vi "S4GUI.vi"(7 "Tab ObsEng":enum32{"Obs", "CCD modes", "Guider", "Eng"}(tab)) -> ()   [LabVIEW 2018] (continued)
            n3354 = call "Write AcquisitionB.vi"("error in (no error)"=w7300, "Acquisition.lvclass"=w7299, "S4ACS_GUI in"=w7297) -> ("error out"=w7303:errorcluster, "S4ACS_GUI out"=w7304:refnum<class "S4GUI.lvclass">)  [unwired: 7 in]
          }
          frame #2 {
            # "object"
            # "suffix"
            # "obsType"
            n3355 = call-dynamic "Read AcquisitionC.vi"("error in (no error)"=w7354, "S4ACS_GUI in"=w7355) -> ("error out"=w7347:errorcluster, "Acquisition.lvclass"=w7346:refnum<class "Acquisition.lvclass">, "S4ACS_GUI out"=w7341:refnum<class "S4GUI.lvclass">)  [unwired: 7 in]
            n3356 = call-dynamic "Read Channel.vi"("error in (no error)"=w7347, "Acquisition in"=w7346) -> ("error out"=w7320:errorcluster, "Channel.lvclass"=w7322:refnum<class "Channel.lvclass">, "Acquisition out"=w7340:refnum<class "Acquisition.lvclass">)  [unwired: 7 in]
            n3357 = local read "Filter3"() -> (w7323:u8)
            n3358 = call-dynamic "Write Filter.vi"("error in (no error)"=w7320, "Filter"=w7323, "Channel in"=w7322) -> ("error out"=w7319:errorcluster, "Channel out"=w7321:refnum<class "Channel.lvclass">)  [unwired: 7 in]
            n3359 = call-dynamic "Read Interface.vi"("error in (no error)"=w7319, "Channel in"=w7321) -> ("error out"=w7332:errorcluster, "Interface.lvclass"=w7333:refnum<class "Interface.lvclass">, "Channel out"=w7345:refnum<class "Channel.lvclass">)  [unwired: 7 in]
            n3360 = call-dynamic "Write Suffix.vi"("error in (no error)"=w7332, "Suffix"=w7351, "Interface in"=w7333) -> ("error out"=w7350:errorcluster, "Interface out"=w7344:refnum<class "Interface.lvclass">)  [unwired: 7 in]
            n3361 = call-dynamic "Write ObsType.vi"("error in (no error)"=w7350, "ObsType"=w7336, "Interface in"=w7344) -> ("error out"=w7349:errorcluster, "Interface out"=w7343:refnum<class "Interface.lvclass">)  [unwired: 7 in]
            n3362 = call-dynamic "Write Object.vi"("error in (no error)"=w7349, "Object"=w7335, "Interface in"=w7343) -> ("error out"=w7348:errorcluster, "Interface out"=w7342:refnum<class "Interface.lvclass">)  [unwired: 7 in]
            n3363 = call-dynamic "Write Comments.vi"("error in (no error)"=w7348, "Comments"=w7337, "Interface in"=w7342) -> ("error out"=w7329:errorcluster, "Interface out"=w7328:refnum<class "Interface.lvclass">)  [unwired: 7 in]
            n3364 = call-dynamic "Write Observer.vi"("error in (no error)"=w7329, "Observer"=w7334, "Interface in"=w7328) -> ("error out"=w7330:errorcluster, "Interface out"=w7331:refnum<class "Interface.lvclass">)  [unwired: 7 in]
            n3365 = call-dynamic "Write Interface.vi"("error in (no error)"=w7330, "Interface.lvclass"=w7331, "Channel in"=w7345) -> ("error out"=w7326:errorcluster, "Channel out"=w7327:refnum<class "Channel.lvclass">)  [unwired: 7 in]
            n3366 = disable-structure shown="Enabled" {
              disable-tunnel: w7327 -> [w7362 w7367]
              disable-tunnel: w7326 -> [w7361 w7366]
              disable-tunnel: [w7359 w7367] -> w7325
              disable-tunnel: [w7356 w7366] -> w7324
              frame Disabled {
                n3367 = call-dynamic "Read State Machine.vi"("error in (no error)"=w7361, "Device in"=w7362) -> ("error out"=w7365:errorcluster, "State Machine.lvclass"=w7358:refnum<class "State Machine.lvclass">, "Device out"=w7360:refnum<class "Channel.lvclass">)  [unwired: 7 in]
                n3368 = call "Next State.vi"("error in (no error)"=w7365, "New_State"=12, "State Machine in"=w7358) -> ("error out"=w7364:errorcluster, "State Machine out"=w7357:refnum<class "State Machine.lvclass">)  [unwired: 7 in]
                n3369 = call-dynamic "Write State Machine.vi"("error in (no error)"=w7364, "State Machine.lvclass"=w7357, "Device in"=w7360) -> ("error out"=w7356:errorcluster, "Device out"=w7359:refnum<class "Channel.lvclass">)  [unwired: 7 in]
              }
              frame Enabled {
              }
            }
            n3370 = call-dynamic "Write Channel.vi"("error in (no error)"=w7324, "Channel.lvclass"=w7325, "Acquisition in"=w7340) -> ("error out"=w7338:errorcluster, "Acquisition out"=w7339:refnum<class "Acquisition.lvclass">)  [unwired: 7 in]
            n3371 = call-dynamic "Write AcquisitionC.vi"("error in (no error)"=w7338, "Acquisition.lvclass"=w7339, "S4ACS_GUI in"=w7341) -> ("error out"=w7352:errorcluster, "S4ACS_GUI out"=w7353:refnum<class "S4GUI.lvclass">)  [unwired: 7 in]
          }
          frame #3 {
            # "object"
            # "suffix"
            # "obsType"
            n3372 = call-dynamic "Read AcquisitionD.vi"("error in (no error)"=w7403, "S4ACS_GUI in"=w7404) -> ("error out"=w7396:errorcluster, "Acquisition.lvclass"=w7395:refnum<class "Acquisition.lvclass">, "S4ACS_GUI out"=w7390:refnum<class "S4GUI.lvclass">)  [unwired: 7 in]
            n3373 = call-dynamic "Read Channel.vi"("error in (no error)"=w7396, "Acquisition in"=w7395) -> ("error out"=w7369:errorcluster, "Channel.lvclass"=w7371:refnum<class "Channel.lvclass">, "Acquisition out"=w7389:refnum<class "Acquisition.lvclass">)  [unwired: 7 in]
            n3374 = local read "Filter4"() -> (w7372:u8)
            n3375 = call-dynamic "Write Filter.vi"("error in (no error)"=w7369, "Filter"=w7372, "Channel in"=w7371) -> ("error out"=w7368:errorcluster, "Channel out"=w7370:refnum<class "Channel.lvclass">)  [unwired: 7 in]
            n3376 = call-dynamic "Read Interface.vi"("error in (no error)"=w7368, "Channel in"=w7370) -> ("error out"=w7381:errorcluster, "Interface.lvclass"=w7382:refnum<class "Interface.lvclass">, "Channel out"=w7394:refnum<class "Channel.lvclass">)  [unwired: 7 in]
            n3377 = call-dynamic "Write Suffix.vi"("error in (no error)"=w7381, "Suffix"=w7400, "Interface in"=w7382) -> ("error out"=w7399:errorcluster, "Interface out"=w7393:refnum<class "Interface.lvclass">)  [unwired: 7 in]
            n3378 = call-dynamic "Write ObsType.vi"("error in (no error)"=w7399, "ObsType"=w7385, "Interface in"=w7393) -> ("error out"=w7398:errorcluster, "Interface out"=w7392:refnum<class "Interface.lvclass">)  [unwired: 7 in]
            n3379 = call-dynamic "Write Object.vi"("error in (no error)"=w7398, "Object"=w7384, "Interface in"=w7392) -> ("error out"=w7397:errorcluster, "Interface out"=w7391:refnum<class "Interface.lvclass">)  [unwired: 7 in]
            n3380 = call-dynamic "Write Comments.vi"("error in (no error)"=w7397, "Comments"=w7386, "Interface in"=w7391) -> ("error out"=w7380:errorcluster, "Interface out"=w7379:refnum<class "Interface.lvclass">)  [unwired: 7 in]
            n3381 = call-dynamic "Write Observer.vi"("error in (no error)"=w7380, "Observer"=w7383, "Interface in"=w7379) -> ("error out"=w7378:errorcluster, "Interface out"=w7377:refnum<class "Interface.lvclass">)  [unwired: 7 in]
            n3382 = call-dynamic "Write Interface.vi"("error in (no error)"=w7378, "Interface.lvclass"=w7377, "Channel in"=w7394) -> ("error out"=w7374:errorcluster, "Channel out"=w7376:refnum<class "Channel.lvclass">)  [unwired: 7 in]
            n3383 = disable-structure shown="Enabled" {
              disable-tunnel: w7376 -> [w7411 w7416]
              disable-tunnel: [w7409 w7416] -> w7375
              disable-tunnel: w7374 -> [w7408 w7415]
              disable-tunnel: [w7407 w7415] -> w7373
              frame Disabled {
                n3384 = call-dynamic "Read State Machine.vi"("error in (no error)"=w7408, "Device in"=w7411) -> ("error out"=w7414:errorcluster, "State Machine.lvclass"=w7406:refnum<class "State Machine.lvclass">, "Device out"=w7410:refnum<class "Channel.lvclass">)  [unwired: 7 in]
                n3385 = call "Next State.vi"("error in (no error)"=w7414, "New_State"=12, "State Machine in"=w7406) -> ("error out"=w7413:errorcluster, "State Machine out"=w7405:refnum<class "State Machine.lvclass">)  [unwired: 7 in]
                n3386 = call-dynamic "Write State Machine.vi"("error in (no error)"=w7413, "State Machine.lvclass"=w7405, "Device in"=w7410) -> ("error out"=w7407:errorcluster, "Device out"=w7409:refnum<class "Channel.lvclass">)  [unwired: 7 in]
              }
              frame Enabled {
              }
            }
            n3387 = call-dynamic "Write Channel.vi"("error in (no error)"=w7373, "Channel.lvclass"=w7375, "Acquisition in"=w7389) -> ("error out"=w7387:errorcluster, "Acquisition out"=w7388:refnum<class "Acquisition.lvclass">)  [unwired: 7 in]
            n3388 = call-dynamic "Write AcquisitionD.vi"("error in (no error)"=w7387, "Acquisition.lvclass"=w7388, "S4ACS_GUI in"=w7390) -> ("error out"=w7401:errorcluster, "S4ACS_GUI out"=w7402:refnum<class "S4GUI.lvclass">)  [unwired: 7 in]
          }
        }
      }
      event "DFLAT Comments", "SFLAT Comments", "DARK Comments", "ZERO Comments", "FOCUS Comments", "OBJECT Comments": Value Change {
        n3389 = event-data() -> ("NewVal"=w7417:string)  [unwired: 1 in, 5 out]
        n3390 = disable-structure shown="Enabled" {
          disable-tunnel: w7425 -> [w7434 w7608]
          disable-tunnel: w7424 -> [w7433 w7607]
          disable-tunnel: w7423 -> [w7432 _]
          disable-tunnel: w7422 -> [w7431 _]
          disable-tunnel: w7421 -> [w7430 _]
          disable-tunnel: w7420 -> [w7429 _]
          disable-tunnel: [w7428 w7608] -> w7419
          disable-tunnel: [w7427 w7607] -> w7418
          disable-tunnel: w7417 -> [w7426 _]
          frame Disabled {
            n3391 = stacked-sequence {
              seq-local: [w7462 _ _ _] -> [_ w7520 _ _]
              seq-local: [w7461 _ _ _] -> [_ w7519 _ _]
              seq-local: [_ w7518 _ _] -> [_ _ w7563 _]
              seq-local: [_ w7517 _ _] -> [_ _ w7562 _]
              seq-local: [_ _ w7561 _] -> [_ _ _ w7606]
              seq-local: [_ _ w7560 _] -> [_ _ _ w7605]
              tunnel: w7433 -> [w7474 _ _ _]
              tunnel: w7434 -> [w7473 _ _ _]
              tunnel: [_ _ _ w7604] -> w7428
              tunnel: [_ _ _ w7603] -> w7427
              tunnel: w7431 -> [w7460 w7516 w7559 w7602]
              tunnel: w7426 -> [w7459 w7515 w7545 w7588]
              tunnel: w7429 -> [w7458 w7501 w7544 w7587]
              tunnel: w7432 -> [w7457 w7500 w7543 w7586]
              tunnel: w7430 -> [w7456 w7499 w7542 w7585]
              frame #0 {
                # "observer"
                # "comment"
                # "object"
                # "suffix"
                # "obsType"
                n3392 = call-dynamic "Read AcquisitionA.vi"("error in (no error)"=w7474, "S4ACS_GUI in"=w7473) -> ("error out"=w7472:errorcluster, "Acquisition.lvclass"=w7471:refnum<class "Acquisition.lvclass">, "S4ACS_GUI out"=w7466:refnum<class "S4GUI.lvclass">)  [unwired: 7 in]
                n3393 = call-dynamic "Read Channel.vi"("error in (no error)"=w7472, "Acquisition in"=w7471) -> ("error out"=w7436:errorcluster, "Channel.lvclass"=w7439:refnum<class "Channel.lvclass">, "Acquisition out"=w7465:refnum<class "Acquisition.lvclass">)  [unwired: 7 in]
                n3394 = local read "Filter1"() -> (w7437:u8)
                n3395 = call-dynamic "Write Filter.vi"("error in (no error)"=w7436, "Filter"=w7437, "Channel in"=w7439) -> ("error out"=w7435:errorcluster, "Channel out"=w7438:refnum<class "Channel.lvclass">)  [unwired: 7 in]
                n3396 = call-dynamic "Read Interface.vi"("error in (no error)"=w7435, "Channel in"=w7438) -> ("error out"=w7452:errorcluster, "Interface.lvclass"=w7453:refnum<class "Interface.lvclass">, "Channel out"=w7470:refnum<class "Channel.lvclass">)  [unwired: 7 in]
                n3397 = call-dynamic "Write Suffix.vi"("error in (no error)"=w7452, "Suffix"=w7460, "Interface in"=w7453) -> ("error out"=w7477:errorcluster, "Interface out"=w7469:refnum<class "Interface.lvclass">)  [unwired: 7 in]
                n3398 = call-dynamic "Write ObsType.vi"("error in (no error)"=w7477, "ObsType"=w7458, "Interface in"=w7469) -> ("error out"=w7476:errorcluster, "Interface out"=w7468:refnum<class "Interface.lvclass">)  [unwired: 7 in]
                n3399 = call-dynamic "Write Object.vi"("error in (no error)"=w7476, "Object"=w7457, "Interface in"=w7468) -> ("error out"=w7475:errorcluster, "Interface out"=w7467:refnum<class "Interface.lvclass">)  [unwired: 7 in]
                n3400 = call-dynamic "Write Comments.vi"("error in (no error)"=w7475, "Comments"=w7459, "Interface in"=w7467) -> ("error out"=w7455:errorcluster, "Interface out"=w7454:refnum<class "Interface.lvclass">)  [unwired: 7 in]
                n3401 = call-dynamic "Write Observer.vi"("error in (no error)"=w7455, "Observer"=w7456, "Interface in"=w7454) -> ("error out"=w7450:errorcluster, "Interface out"=w7451:refnum<class "Interface.lvclass">)  [unwired: 7 in]
                n3402 = call-dynamic "Write Interface.vi"("error in (no error)"=w7450, "Interface.lvclass"=w7451, "Channel in"=w7470) -> ("error out"=w7446:errorcluster, "Channel out"=w7449:refnum<class "Channel.lvclass">)  [unwired: 7 in]
                n3403 = call-dynamic "Read State Machine.vi"("error in (no error)"=w7446, "Device in"=w7449) -> ("error out"=w7445:errorcluster, "State Machine.lvclass"=w7443:refnum<class "State Machine.lvclass">, "Device out"=w7448:refnum<class "Channel.lvclass">)  [unwired: 7 in]
                n3404 = call "Next State.vi"("error in (no error)"=w7445, "New_State"=12, "State Machine in"=w7443) -> ("error out"=w7444:errorcluster, "State Machine out"=w7442:refnum<class "State Machine.lvclass">)  [unwired: 7 in]
                n3405 = call-dynamic "Write State Machine.vi"("error in (no error)"=w7444, "State Machine.lvclass"=w7442, "Device in"=w7448) -> ("error out"=w7441:errorcluster, "Device out"=w7447:refnum<class "Channel.lvclass">)  [unwired: 7 in]
                n3406 = call-dynamic "Write Channel.vi"("error in (no error)"=w7441, "Channel.lvclass"=w7447, "Acquisition in"=w7465) -> ("error out"=w7463:errorcluster, "Acquisition out"=w7464:refnum<class "Acquisition.lvclass">)  [unwired: 7 in]
                n3407 = call-dynamic "Write AcquisitionA.vi"("error in (no error)"=w7463, "Acquisition.lvclass"=w7464, "S4ACS_GUI in"=w7466) -> ("error out"=w7461:errorcluster, "S4ACS_GUI out"=w7462:refnum<class "S4GUI.lvclass">)  [unwired: 7 in]
              }
              frame #1 {
                # "object"
                # "suffix"
                # "obsType"
                n3408 = call "Read AcquisitionB.vi"("error in (no error)"=w7519, "S4ACS_GUI in"=w7520) -> ("error out"=w7505:errorcluster, "Acquisition.lvclass"=w7506:refnum<class "Acquisition.lvclass">, "S4ACS_GUI out"=w7511:refnum<class "S4GUI.lvclass">)  [unwired: 7 in]
                n3409 = call-dynamic "Read Channel.vi"("error in (no error)"=w7505, "Acquisition in"=w7506) -> ("error out"=w7479:errorcluster, "Channel.lvclass"=w7481:refnum<class "Channel.lvclass">, "Acquisition out"=w7512:refnum<class "Acquisition.lvclass">)  [unwired: 7 in]
                n3410 = local read "Filter2"() -> (w7482:u8)
                n3411 = call-dynamic "Write Filter.vi"("error in (no error)"=w7479, "Filter"=w7482, "Channel in"=w7481) -> ("error out"=w7478:errorcluster, "Channel out"=w7480:refnum<class "Channel.lvclass">)  [unwired: 7 in]
                n3412 = call-dynamic "Read Interface.vi"("error in (no error)"=w7478, "Channel in"=w7480) -> ("error out"=w7493:errorcluster, "Interface.lvclass"=w7494:refnum<class "Interface.lvclass">, "Channel out"=w7507:refnum<class "Channel.lvclass">)  [unwired: 7 in]
                n3413 = call-dynamic "Write Suffix.vi"("error in (no error)"=w7493, "Suffix"=w7516, "Interface in"=w7494) -> ("error out"=w7502:errorcluster, "Interface out"=w7508:refnum<class "Interface.lvclass">)  [unwired: 7 in]
                n3414 = call-dynamic "Write ObsType.vi"("error in (no error)"=w7502, "ObsType"=w7501, "Interface in"=w7508) -> ("error out"=w7503:errorcluster, "Interface out"=w7509:refnum<class "Interface.lvclass">)  [unwired: 7 in]
                n3415 = call-dynamic "Write Object.vi"("error in (no error)"=w7503, "Object"=w7500, "Interface in"=w7509) -> ("error out"=w7504:errorcluster, "Interface out"=w7510:refnum<class "Interface.lvclass">)  [unwired: 7 in]
                n3416 = call-dynamic "Write Comments.vi"("error in (no error)"=w7504, "Comments"=w7515, "Interface in"=w7510) -> ("error out"=w7496:errorcluster, "Interface out"=w7495:refnum<class "Interface.lvclass">)  [unwired: 7 in]
                n3417 = call-dynamic "Write Observer.vi"("error in (no error)"=w7496, "Observer"=w7499, "Interface in"=w7495) -> ("error out"=w7497:errorcluster, "Interface out"=w7498:refnum<class "Interface.lvclass">)  [unwired: 7 in]
                n3418 = call-dynamic "Write Interface.vi"("error in (no error)"=w7497, "Interface.lvclass"=w7498, "Channel in"=w7507) -> ("error out"=w7486:errorcluster, "Channel out"=w7487:refnum<class "Channel.lvclass">)  [unwired: 7 in]
                n3419 = call-dynamic "Read State Machine.vi"("error in (no error)"=w7486, "Device in"=w7487) -> ("error out"=w7492:errorcluster, "State Machine.lvclass"=w7490:refnum<class "State Machine.lvclass">, "Device out"=w7485:refnum<class "Channel.lvclass">)  [unwired: 7 in]
                n3420 = call "Next State.vi"("error in (no error)"=w7492, "New_State"=12, "State Machine in"=w7490) -> ("error out"=w7491:errorcluster, "State Machine out"=w7489:refnum<class "State Machine.lvclass">)  [unwired: 7 in]
                n3421 = call-dynamic "Write State Machine.vi"("error in (no error)"=w7491, "State Machine.lvclass"=w7489, "Device in"=w7485) -> ("error out"=w7483:errorcluster, "Device out"=w7484:refnum<class "Channel.lvclass">)  [unwired: 7 in]
                n3422 = call-dynamic "Write Channel.vi"("error in (no error)"=w7483, "Channel.lvclass"=w7484, "Acquisition in"=w7512) -> ("error out"=w7514:errorcluster, "Acquisition out"=w7513:refnum<class "Acquisition.lvclass">)  [unwired: 7 in]
                n3423 = call "Write AcquisitionB.vi"("error in (no error)"=w7514, "Acquisition.lvclass"=w7513, "S4ACS_GUI in"=w7511) -> ("error out"=w7517:errorcluster, "S4ACS_GUI out"=w7518:refnum<class "S4GUI.lvclass">)  [unwired: 7 in]
              }
              frame #2 {
                # "object"
                # "suffix"
                # "obsType"
                n3424 = call-dynamic "Read AcquisitionC.vi"("error in (no error)"=w7562, "S4ACS_GUI in"=w7563) -> ("error out"=w7555:errorcluster, "Acquisition.lvclass"=w7554:refnum<class "Acquisition.lvclass">, "S4ACS_GUI out"=w7549:refnum<class "S4GUI.lvclass">)  [unwired: 7 in]
                n3425 = call-dynamic "Read Channel.vi"("error in (no error)"=w7555, "Acquisition in"=w7554) -> ("error out"=w7522:errorcluster, "Channel.lvclass"=w7524:refnum<class "Channel.lvclass">, "Acquisition out"=w7548:refnum<class "Acquisition.lvclass">)  [unwired: 7 in]
                n3426 = local read "Filter3"() -> (w7525:u8)
                n3427 = call-dynamic "Write Filter.vi"("error in (no error)"=w7522, "Filter"=w7525, "Channel in"=w7524) -> ("error out"=w7521:errorcluster, "Channel out"=w7523:refnum<class "Channel.lvclass">)  [unwired: 7 in]
                n3428 = call-dynamic "Read Interface.vi"("error in (no error)"=w7521, "Channel in"=w7523) -> ("error out"=w7540:errorcluster, "Interface.lvclass"=w7541:refnum<class "Interface.lvclass">, "Channel out"=w7553:refnum<class "Channel.lvclass">)  [unwired: 7 in]
                n3429 = call-dynamic "Write Suffix.vi"("error in (no error)"=w7540, "Suffix"=w7559, "Interface in"=w7541) -> ("error out"=w7558:errorcluster, "Interface out"=w7552:refnum<class "Interface.lvclass">)  [unwired: 7 in]
                n3430 = call-dynamic "Write ObsType.vi"("error in (no error)"=w7558, "ObsType"=w7544, "Interface in"=w7552) -> ("error out"=w7557:errorcluster, "Interface out"=w7551:refnum<class "Interface.lvclass">)  [unwired: 7 in]
                n3431 = call-dynamic "Write Object.vi"("error in (no error)"=w7557, "Object"=w7543, "Interface in"=w7551) -> ("error out"=w7556:errorcluster, "Interface out"=w7550:refnum<class "Interface.lvclass">)  [unwired: 7 in]
                n3432 = call-dynamic "Write Comments.vi"("error in (no error)"=w7556, "Comments"=w7545, "Interface in"=w7550) -> ("error out"=w7537:errorcluster, "Interface out"=w7536:refnum<class "Interface.lvclass">)  [unwired: 7 in]
                n3433 = call-dynamic "Write Observer.vi"("error in (no error)"=w7537, "Observer"=w7542, "Interface in"=w7536) -> ("error out"=w7538:errorcluster, "Interface out"=w7539:refnum<class "Interface.lvclass">)  [unwired: 7 in]
                n3434 = call-dynamic "Write Interface.vi"("error in (no error)"=w7538, "Interface.lvclass"=w7539, "Channel in"=w7553) -> ("error out"=w7531:errorcluster, "Channel out"=w7532:refnum<class "Channel.lvclass">)  [unwired: 7 in]
                n3435 = call-dynamic "Read State Machine.vi"("error in (no error)"=w7531, "Device in"=w7532) -> ("error out"=w7535:errorcluster, "State Machine.lvclass"=w7528:refnum<class "State Machine.lvclass">, "Device out"=w7530:refnum<class "Channel.lvclass">)  [unwired: 7 in]
                n3436 = call "Next State.vi"("error in (no error)"=w7535, "New_State"=12, "State Machine in"=w7528) -> ("error out"=w7534:errorcluster, "State Machine out"=w7527:refnum<class "State Machine.lvclass">)  [unwired: 7 in]
                n3437 = call-dynamic "Write State Machine.vi"("error in (no error)"=w7534, "State Machine.lvclass"=w7527, "Device in"=w7530) -> ("error out"=w7526:errorcluster, "Device out"=w7529:refnum<class "Channel.lvclass">)  [unwired: 7 in]
                n3438 = call-dynamic "Write Channel.vi"("error in (no error)"=w7526, "Channel.lvclass"=w7529, "Acquisition in"=w7548) -> ("error out"=w7546:errorcluster, "Acquisition out"=w7547:refnum<class "Acquisition.lvclass">)  [unwired: 7 in]
                n3439 = call-dynamic "Write AcquisitionC.vi"("error in (no error)"=w7546, "Acquisition.lvclass"=w7547, "S4ACS_GUI in"=w7549) -> ("error out"=w7560:errorcluster, "S4ACS_GUI out"=w7561:refnum<class "S4GUI.lvclass">)  [unwired: 7 in]
              }
              frame #3 {
                # "object"
                # "suffix"
                # "obsType"
                n3440 = call-dynamic "Read AcquisitionD.vi"("error in (no error)"=w7605, "S4ACS_GUI in"=w7606) -> ("error out"=w7598:errorcluster, "Acquisition.lvclass"=w7597:refnum<class "Acquisition.lvclass">, "S4ACS_GUI out"=w7592:refnum<class "S4GUI.lvclass">)  [unwired: 7 in]
                n3441 = call-dynamic "Read Channel.vi"("error in (no error)"=w7598, "Acquisition in"=w7597) -> ("error out"=w7565:errorcluster, "Channel.lvclass"=w7567:refnum<class "Channel.lvclass">, "Acquisition out"=w7591:refnum<class "Acquisition.lvclass">)  [unwired: 7 in]
                n3442 = local read "Filter4"() -> (w7568:u8)
                n3443 = call-dynamic "Write Filter.vi"("error in (no error)"=w7565, "Filter"=w7568, "Channel in"=w7567) -> ("error out"=w7564:errorcluster, "Channel out"=w7566:refnum<class "Channel.lvclass">)  [unwired: 7 in]
                n3444 = call-dynamic "Read Interface.vi"("error in (no error)"=w7564, "Channel in"=w7566) -> ("error out"=w7583:errorcluster, "Interface.lvclass"=w7584:refnum<class "Interface.lvclass">, "Channel out"=w7596:refnum<class "Channel.lvclass">)  [unwired: 7 in]
                n3445 = call-dynamic "Write Suffix.vi"("error in (no error)"=w7583, "Suffix"=w7602, "Interface in"=w7584) -> ("error out"=w7601:errorcluster, "Interface out"=w7595:refnum<class "Interface.lvclass">)  [unwired: 7 in]
                n3446 = call-dynamic "Write ObsType.vi"("error in (no error)"=w7601, "ObsType"=w7587, "Interface in"=w7595) -> ("error out"=w7600:errorcluster, "Interface out"=w7594:refnum<class "Interface.lvclass">)  [unwired: 7 in]
                n3447 = call-dynamic "Write Object.vi"("error in (no error)"=w7600, "Object"=w7586, "Interface in"=w7594) -> ("error out"=w7599:errorcluster, "Interface out"=w7593:refnum<class "Interface.lvclass">)  [unwired: 7 in]
                n3448 = call-dynamic "Write Comments.vi"("error in (no error)"=w7599, "Comments"=w7588, "Interface in"=w7593) -> ("error out"=w7582:errorcluster, "Interface out"=w7581:refnum<class "Interface.lvclass">)  [unwired: 7 in]
                n3449 = call-dynamic "Write Observer.vi"("error in (no error)"=w7582, "Observer"=w7585, "Interface in"=w7581) -> ("error out"=w7577:errorcluster, "Interface out"=w7576:refnum<class "Interface.lvclass">)  [unwired: 7 in]
                n3450 = call-dynamic "Write Interface.vi"("error in (no error)"=w7577, "Interface.lvclass"=w7576, "Channel in"=w7596) -> ("error out"=w7572:errorcluster, "Channel out"=w7575:refnum<class "Channel.lvclass">)  [unwired: 7 in]
                n3451 = call-dynamic "Read State Machine.vi"("error in (no error)"=w7572, "Device in"=w7575) -> ("error out"=w7580:errorcluster, "State Machine.lvclass"=w7570:refnum<class "State Machine.lvclass">, "Device out"=w7574:refnum<class "Channel.lvclass">)  [unwired: 7 in]
                n3452 = call "Next State.vi"("error in (no error)"=w7580, "New_State"=12, "State Machine in"=w7570) -> ("error out"=w7579:errorcluster, "State Machine out"=w7569:refnum<class "State Machine.lvclass">)  [unwired: 7 in]
                n3453 = call-dynamic "Write State Machine.vi"("error in (no error)"=w7579, "State Machine.lvclass"=w7569, "Device in"=w7574) -> ("error out"=w7571:errorcluster, "Device out"=w7573:refnum<class "Channel.lvclass">)  [unwired: 7 in]
                n3454 = call-dynamic "Write Channel.vi"("error in (no error)"=w7571, "Channel.lvclass"=w7573, "Acquisition in"=w7591) -> ("error out"=w7589:errorcluster, "Acquisition out"=w7590:refnum<class "Acquisition.lvclass">)  [unwired: 7 in]
                n3455 = call-dynamic "Write AcquisitionD.vi"("error in (no error)"=w7589, "Acquisition.lvclass"=w7590, "S4ACS_GUI in"=w7592) -> ("error out"=w7603:errorcluster, "S4ACS_GUI out"=w7604:refnum<class "S4GUI.lvclass">)  [unwired: 7 in]
              }
            }
          }
          frame Enabled {
          }
        }
      }
      event "object suffix", "dflat suffix", "sflat suffix", "dark suffix", "zero suffix", "focus suffix": Value Change {
        w7609 = T33 0 items=["both", "start of string", "end of string"] ("location (both)")
        # "Remove todos <\\n> e <space> do sufixo:"
        n3456 = event-data() -> ("NewVal"=w7623:string)  [unwired: 1 in, 5 out]
        n3457 = To Lower Case(string=w7623) -> (all lower case string=w7622:string)
        n3458 = call <vilib>:"Trim Whitespace.vi"("string"=w7622, "location (both)"=w7609) -> ("trimmed string"=w7621:string)
        n3459 = Search and Replace String(replace all?=TRUE ("replace all? (F)"), input string=w7621, search string="\n") -> (result string=w7620:string)  [unwired: 5 in, 3 out]
        n3460 = call <vilib>:"Space Constant.vi"() -> ("String"=w7618:string)
        n3461 = Search and Replace String(replace all?=TRUE ("replace all? (F)"), input string=w7620, search string=w7618) -> (result string=w7614:string)  [unwired: 5 in, 3 out]
        n3462 = case shown="\"DARK\"" w7615 {
          tunnel: w7614 -> [w7837 w7844 w7849 w7854 w7859 w7864]
          tunnel: w7613 -> [w7841 w7846 w7851 w7856 w7861 w7866]
          tunnel: w7612 -> [w7839 w7845 w7850 w7855 w7860 w7865]
          tunnel: [w7840 w7843 w7848 w7852 w7857 w7862] -> w7611
          tunnel: [w7838 w7842 w7847 w7853 w7858 w7863] -> w7610
          frame "OBJECT", Default {
            n3463 = local write "object suffix"(w7837) -> ()
            n3464 = call-dynamic "Write object_suffix.vi"("error in (no error)"=w7839, "object"=w7837, "S4GUI in"=w7841) -> ("error out"=w7838:errorcluster, "S4GUI out"=w7840:refnum<class "S4GUI.lvclass">)  [unwired: 7 in]
          }
          frame "DFLAT" {
            n3465 = local write "dflat suffix"(w7844) -> ()
            n3466 = call-dynamic "Write dflat_suffix.vi"("error in (no error)"=w7845, "dflat"=w7844, "S4GUI in"=w7846) -> ("error out"=w7842:errorcluster, "S4GUI out"=w7843:refnum<class "S4GUI.lvclass">)  [unwired: 7 in]
          }
          frame "SFLAT" {
            n3467 = local write "sflat suffix"(w7849) -> ()
            n3468 = call-dynamic "Write sflat_suffix.vi"("error in (no error)"=w7850, "sflat"=w7849, "S4GUI in"=w7851) -> ("error out"=w7847:errorcluster, "S4GUI out"=w7848:refnum<class "S4GUI.lvclass">)  [unwired: 7 in]
          }
          frame "DARK" {
            n3469 = local write "dark suffix"(w7854) -> ()
            n3470 = call-dynamic "Write dark_suffix.vi"("error in (no error)"=w7855, "dark"=w7854, "S4GUI in"=w7856) -> ("error out"=w7853:errorcluster, "S4GUI out"=w7852:refnum<class "S4GUI.lvclass">)  [unwired: 7 in]
          }
          frame "ZERO" {
            n3471 = local write "zero suffix"(w7859) -> ()
            n3472 = call-dynamic "Write zero_suffix.vi"("error in (no error)"=w7860, "zero"=w7859, "S4GUI in"=w7861) -> ("error out"=w7858:errorcluster, "S4GUI out"=w7857:refnum<class "S4GUI.lvclass">)  [unwired: 7 in]
          }
          frame "FOCUS" {
            n3473 = local write "focus suffix"(w7864) -> ()
            n3474 = call-dynamic "Write focus_suffix.vi"("error in (no error)"=w7865, "focus"=w7864, "S4GUI in"=w7866) -> ("error out"=w7863:errorcluster, "S4GUI out"=w7862:refnum<class "S4GUI.lvclass">)  [unwired: 7 in]
          }
        }
        n3475 = disable-structure shown="Enabled" {
          disable-tunnel: w7629 -> [w7638 _]
          disable-tunnel: w7628 -> [w7637 _]
          disable-tunnel: w7627 -> [w7636 _]
          disable-tunnel: w7626 -> [w7635 _]
          disable-tunnel: [w7634 w7836] -> w7625
          disable-tunnel: [w7633 w7835] -> w7624
          disable-tunnel: w7614 -> [w7632 _]
          disable-tunnel: w7611 -> [w7631 w7836]
          disable-tunnel: w7610 -> [w7630 w7835]
          frame Disabled {
            n3476 = stacked-sequence {
              seq-local: [w7660 _ _ _] -> [_ w7724 _ _]
              seq-local: [w7659 _ _ _] -> [_ w7723 _ _]
              seq-local: [_ w7722 _ _] -> [_ _ w7773 _]
              seq-local: [_ w7721 _ _] -> [_ _ w7772 _]
              seq-local: [_ _ w7771 _] -> [_ _ _ w7822]
              seq-local: [_ _ w7770 _] -> [_ _ _ w7821]
              tunnel: w7630 -> [w7672 _ _ _]
              tunnel: w7631 -> [w7671 _ _ _]
              tunnel: [_ _ _ w7820] -> w7634
              tunnel: [_ _ _ w7819] -> w7633
              tunnel: w7632 -> [w7658 w7720 w7769 w7818]
              tunnel: w7637 -> [w7657 w7719 w7755 w7804]
              tunnel: w7635 -> [w7656 w7705 w7754 w7803]
              tunnel: w7638 -> [w7655 w7704 w7753 w7802]
              tunnel: w7636 -> [w7654 w7703 w7752 w7801]
              frame #0 {
                # "observer"
                # "comment"
                # "object"
                # "suffix"
                # "obsType"
                n3477 = call-dynamic "Read AcquisitionA.vi"("error in (no error)"=w7672, "S4ACS_GUI in"=w7671) -> ("error out"=w7670:errorcluster, "Acquisition.lvclass"=w7669:refnum<class "Acquisition.lvclass">, "S4ACS_GUI out"=w7664:refnum<class "S4GUI.lvclass">)  [unwired: 7 in]
                n3478 = call-dynamic "Read Channel.vi"("error in (no error)"=w7670, "Acquisition in"=w7669) -> ("error out"=w7640:errorcluster, "Channel.lvclass"=w7643:refnum<class "Channel.lvclass">, "Acquisition out"=w7663:refnum<class "Acquisition.lvclass">)  [unwired: 7 in]
                n3479 = local read "Filter1"() -> (w7641:u8)
                n3480 = call-dynamic "Write Filter.vi"("error in (no error)"=w7640, "Filter"=w7641, "Channel in"=w7643) -> ("error out"=w7639:errorcluster, "Channel out"=w7642:refnum<class "Channel.lvclass">)  [unwired: 7 in]
                n3481 = call-dynamic "Read Interface.vi"("error in (no error)"=w7639, "Channel in"=w7642) -> ("error out"=w7650:errorcluster, "Interface.lvclass"=w7651:refnum<class "Interface.lvclass">, "Channel out"=w7668:refnum<class "Channel.lvclass">)  [unwired: 7 in]
                n3482 = call-dynamic "Write Suffix.vi"("error in (no error)"=w7650, "Suffix"=w7658, "Interface in"=w7651) -> ("error out"=w7675:errorcluster, "Interface out"=w7667:refnum<class "Interface.lvclass">)  [unwired: 7 in]
                n3483 = call-dynamic "Write ObsType.vi"("error in (no error)"=w7675, "ObsType"=w7656, "Interface in"=w7667) -> ("error out"=w7674:errorcluster, "Interface out"=w7666:refnum<class "Interface.lvclass">)  [unwired: 7 in]
                n3484 = call-dynamic "Write Object.vi"("error in (no error)"=w7674, "Object"=w7655, "Interface in"=w7666) -> ("error out"=w7673:errorcluster, "Interface out"=w7665:refnum<class "Interface.lvclass">)  [unwired: 7 in]
                n3485 = call-dynamic "Write Comments.vi"("error in (no error)"=w7673, "Comments"=w7657, "Interface in"=w7665) -> ("error out"=w7653:errorcluster, "Interface out"=w7652:refnum<class "Interface.lvclass">)  [unwired: 7 in]
                n3486 = call-dynamic "Write Observer.vi"("error in (no error)"=w7653, "Observer"=w7654, "Interface in"=w7652) -> ("error out"=w7648:errorcluster, "Interface out"=w7649:refnum<class "Interface.lvclass">)  [unwired: 7 in]
                n3487 = call-dynamic "Write Interface.vi"("error in (no error)"=w7648, "Interface.lvclass"=w7649, "Channel in"=w7668) -> ("error out"=w7645:errorcluster, "Channel out"=w7647:refnum<class "Channel.lvclass">)  [unwired: 7 in]
                n3488 = disable-structure shown="Enabled" {
                  disable-tunnel: w7647 -> [w7685 w7687]
                  disable-tunnel: [w7683 w7687] -> w7646
                  disable-tunnel: w7645 -> [w7682 w7686]
                  disable-tunnel: [w7677 w7686] -> w7644
                  frame Disabled {
                    n3489 = call-dynamic "Read State Machine.vi"("error in (no error)"=w7682, "Device in"=w7685) -> ("error out"=w7681:errorcluster, "State Machine.lvclass"=w7679:refnum<class "State Machine.lvclass">, "Device out"=w7684:refnum<class "Channel.lvclass">)  [unwired: 7 in]
                    n3490 = call "Next State.vi"("error in (no error)"=w7681, "New_State"=12, "State Machine in"=w7679) -> ("error out"=w7680:errorcluster, "State Machine out"=w7678:refnum<class "State Machine.lvclass">)  [unwired: 7 in]
                    n3491 = call-dynamic "Write State Machine.vi"("error in (no error)"=w7680, "State Machine.lvclass"=w7678, "Device in"=w7684) -> ("error out"=w7677:errorcluster, "Device out"=w7683:refnum<class "Channel.lvclass">)  [unwired: 7 in]
                  }
                  frame Enabled {
                  }
                }
                n3492 = call-dynamic "Write Channel.vi"("error in (no error)"=w7644, "Channel.lvclass"=w7646, "Acquisition in"=w7663) -> ("error out"=w7661:errorcluster, "Acquisition out"=w7662:refnum<class "Acquisition.lvclass">)  [unwired: 7 in]
                n3493 = call-dynamic "Write AcquisitionA.vi"("error in (no error)"=w7661, "Acquisition.lvclass"=w7662, "S4ACS_GUI in"=w7664) -> ("error out"=w7659:errorcluster, "S4ACS_GUI out"=w7660:refnum<class "S4GUI.lvclass">)  [unwired: 7 in]
              }
              frame #1 {
                # "object"
                # "suffix"
                # "obsType"
                n3494 = call "Read AcquisitionB.vi"("error in (no error)"=w7723, "S4ACS_GUI in"=w7724) -> ("error out"=w7709:errorcluster, "Acquisition.lvclass"=w7710:refnum<class "Acquisition.lvclass">, "S4ACS_GUI out"=w7715:refnum<class "S4GUI.lvclass">)  [unwired: 7 in]
                n3495 = call-dynamic "Read Channel.vi"("error in (no error)"=w7709, "Acquisition in"=w7710) -> ("error out"=w7689:errorcluster, "Channel.lvclass"=w7691:refnum<class "Channel.lvclass">, "Acquisition out"=w7716:refnum<class "Acquisition.lvclass">)  [unwired: 7 in]
                n3496 = local read "Filter2"() -> (w7692:u8)
                n3497 = call-dynamic "Write Filter.vi"("error in (no error)"=w7689, "Filter"=w7692, "Channel in"=w7691) -> ("error out"=w7688:errorcluster, "Channel out"=w7690:refnum<class "Channel.lvclass">)  [unwired: 7 in]
                n3498 = call-dynamic "Read Interface.vi"("error in (no error)"=w7688, "Channel in"=w7690) -> ("error out"=w7697:errorcluster, "Interface.lvclass"=w7698:refnum<class "Interface.lvclass">, "Channel out"=w7711:refnum<class "Channel.lvclass">)  [unwired: 7 in]
                n3499 = call-dynamic "Write Suffix.vi"("error in (no error)"=w7697, "Suffix"=w7720, "Interface in"=w7698) -> ("error out"=w7706:errorcluster, "Interface out"=w7712:refnum<class "Interface.lvclass">)  [unwired: 7 in]
                n3500 = call-dynamic "Write ObsType.vi"("error in (no error)"=w7706, "ObsType"=w7705, "Interface in"=w7712) -> ("error out"=w7707:errorcluster, "Interface out"=w7713:refnum<class "Interface.lvclass">)  [unwired: 7 in]
                n3501 = call-dynamic "Write Object.vi"("error in (no error)"=w7707, "Object"=w7704, "Interface in"=w7713) -> ("error out"=w7708:errorcluster, "Interface out"=w7714:refnum<class "Interface.lvclass">)  [unwired: 7 in]
                n3502 = call-dynamic "Write Comments.vi"("error in (no error)"=w7708, "Comments"=w7719, "Interface in"=w7714) -> ("error out"=w7700:errorcluster, "Interface out"=w7699:refnum<class "Interface.lvclass">)  [unwired: 7 in]
                n3503 = call-dynamic "Write Observer.vi"("error in (no error)"=w7700, "Observer"=w7703, "Interface in"=w7699) -> ("error out"=w7701:errorcluster, "Interface out"=w7702:refnum<class "Interface.lvclass">)  [unwired: 7 in]
                n3504 = call-dynamic "Write Interface.vi"("error in (no error)"=w7701, "Interface.lvclass"=w7702, "Channel in"=w7711) -> ("error out"=w7695:errorcluster, "Channel out"=w7696:refnum<class "Channel.lvclass">)  [unwired: 7 in]
                n3505 = disable-structure shown="Enabled" {
                  disable-tunnel: w7696 -> [w7729 w7736]
                  disable-tunnel: w7695 -> [w7728 w7735]
                  disable-tunnel: [w7726 w7736] -> w7694
                  disable-tunnel: [w7725 w7735] -> w7693
                  frame Disabled {
                    n3506 = call-dynamic "Read State Machine.vi"("error in (no error)"=w7728, "Device in"=w7729) -> ("error out"=w7734:errorcluster, "State Machine.lvclass"=w7732:refnum<class "State Machine.lvclass">, "Device out"=w7727:refnum<class "Channel.lvclass">)  [unwired: 7 in]
                    n3507 = call "Next State.vi"("error in (no error)"=w7734, "New_State"=12, "State Machine in"=w7732) -> ("error out"=w7733:errorcluster, "State Machine out"=w7731:refnum<class "State Machine.lvclass">)  [unwired: 7 in]
                    n3508 = call-dynamic "Write State Machine.vi"("error in (no error)"=w7733, "State Machine.lvclass"=w7731, "Device in"=w7727) -> ("error out"=w7725:errorcluster, "Device out"=w7726:refnum<class "Channel.lvclass">)  [unwired: 7 in]
                  }
                  frame Enabled {
                  }
                }
                n3509 = call-dynamic "Write Channel.vi"("error in (no error)"=w7693, "Channel.lvclass"=w7694, "Acquisition in"=w7716) -> ("error out"=w7718:errorcluster, "Acquisition out"=w7717:refnum<class "Acquisition.lvclass">)  [unwired: 7 in]
                n3510 = call "Write AcquisitionB.vi"("error in (no error)"=w7718, "Acquisition.lvclass"=w7717, "S4ACS_GUI in"=w7715) -> ("error out"=w7721:errorcluster, "S4ACS_GUI out"=w7722:refnum<class "S4GUI.lvclass">)  [unwired: 7 in]
              }
              frame #2 {
                # "object"
                # "suffix"
                # "obsType"
                n3511 = call-dynamic "Read AcquisitionC.vi"("error in (no error)"=w7772, "S4ACS_GUI in"=w7773) -> ("error out"=w7765:errorcluster, "Acquisition.lvclass"=w7764:refnum<class "Acquisition.lvclass">, "S4ACS_GUI out"=w7759:refnum<class "S4GUI.lvclass">)  [unwired: 7 in]
                n3512 = call-dynamic "Read Channel.vi"("error in (no error)"=w7765, "Acquisition in"=w7764) -> ("error out"=w7738:errorcluster, "Channel.lvclass"=w7740:refnum<class "Channel.lvclass">, "Acquisition out"=w7758:refnum<class "Acquisition.lvclass">)  [unwired: 7 in]
                n3513 = local read "Filter3"() -> (w7741:u8)
                n3514 = call-dynamic "Write Filter.vi"("error in (no error)"=w7738, "Filter"=w7741, "Channel in"=w7740) -> ("error out"=w7737:errorcluster, "Channel out"=w7739:refnum<class "Channel.lvclass">)  [unwired: 7 in]
                n3515 = call-dynamic "Read Interface.vi"("error in (no error)"=w7737, "Channel in"=w7739) -> ("error out"=w7750:errorcluster, "Interface.lvclass"=w7751:refnum<class "Interface.lvclass">, "Channel out"=w7763:refnum<class "Channel.lvclass">)  [unwired: 7 in]
                n3516 = call-dynamic "Write Suffix.vi"("error in (no error)"=w7750, "Suffix"=w7769, "Interface in"=w7751) -> ("error out"=w7768:errorcluster, "Interface out"=w7762:refnum<class "Interface.lvclass">)  [unwired: 7 in]
                n3517 = call-dynamic "Write ObsType.vi"("error in (no error)"=w7768, "ObsType"=w7754, "Interface in"=w7762) -> ("error out"=w7767:errorcluster, "Interface out"=w7761:refnum<class "Interface.lvclass">)  [unwired: 7 in]
                n3518 = call-dynamic "Write Object.vi"("error in (no error)"=w7767, "Object"=w7753, "Interface in"=w7761) -> ("error out"=w7766:errorcluster, "Interface out"=w7760:refnum<class "Interface.lvclass">)  [unwired: 7 in]
                n3519 = call-dynamic "Write Comments.vi"("error in (no error)"=w7766, "Comments"=w7755, "Interface in"=w7760) -> ("error out"=w7747:errorcluster, "Interface out"=w7746:refnum<class "Interface.lvclass">)  [unwired: 7 in]
                n3520 = call-dynamic "Write Observer.vi"("error in (no error)"=w7747, "Observer"=w7752, "Interface in"=w7746) -> ("error out"=w7748:errorcluster, "Interface out"=w7749:refnum<class "Interface.lvclass">)  [unwired: 7 in]
                n3521 = call-dynamic "Write Interface.vi"("error in (no error)"=w7748, "Interface.lvclass"=w7749, "Channel in"=w7763) -> ("error out"=w7744:errorcluster, "Channel out"=w7745:refnum<class "Channel.lvclass">)  [unwired: 7 in]
                n3522 = disable-structure shown="Enabled" {
                  disable-tunnel: w7745 -> [w7780 w7785]
                  disable-tunnel: w7744 -> [w7779 w7784]
                  disable-tunnel: [w7777 w7785] -> w7743
                  disable-tunnel: [w7774 w7784] -> w7742
                  frame Disabled {
                    n3523 = call-dynamic "Read State Machine.vi"("error in (no error)"=w7779, "Device in"=w7780) -> ("error out"=w7783:errorcluster, "State Machine.lvclass"=w7776:refnum<class "State Machine.lvclass">, "Device out"=w7778:refnum<class "Channel.lvclass">)  [unwired: 7 in]
                    n3524 = call "Next State.vi"("error in (no error)"=w7783, "New_State"=12, "State Machine in"=w7776) -> ("error out"=w7782:errorcluster, "State Machine out"=w7775:refnum<class "State Machine.lvclass">)  [unwired: 7 in]
                    n3525 = call-dynamic "Write State Machine.vi"("error in (no error)"=w7782, "State Machine.lvclass"=w7775, "Device in"=w7778) -> ("error out"=w7774:errorcluster, "Device out"=w7777:refnum<class "Channel.lvclass">)  [unwired: 7 in]
                  }
                  frame Enabled {
                  }
                }
                n3526 = call-dynamic "Write Channel.vi"("error in (no error)"=w7742, "Channel.lvclass"=w7743, "Acquisition in"=w7758) -> ("error out"=w7756:errorcluster, "Acquisition out"=w7757:refnum<class "Acquisition.lvclass">)  [unwired: 7 in]
                n3527 = call-dynamic "Write AcquisitionC.vi"("error in (no error)"=w7756, "Acquisition.lvclass"=w7757, "S4ACS_GUI in"=w7759) -> ("error out"=w7770:errorcluster, "S4ACS_GUI out"=w7771:refnum<class "S4GUI.lvclass">)  [unwired: 7 in]
              }
              frame #3 {
                # "object"
                # "suffix"
                # "obsType"
                n3528 = call-dynamic "Read AcquisitionD.vi"("error in (no error)"=w7821, "S4ACS_GUI in"=w7822) -> ("error out"=w7814:errorcluster, "Acquisition.lvclass"=w7813:refnum<class "Acquisition.lvclass">, "S4ACS_GUI out"=w7808:refnum<class "S4GUI.lvclass">)  [unwired: 7 in]
                n3529 = call-dynamic "Read Channel.vi"("error in (no error)"=w7814, "Acquisition in"=w7813) -> ("error out"=w7787:errorcluster, "Channel.lvclass"=w7789:refnum<class "Channel.lvclass">, "Acquisition out"=w7807:refnum<class "Acquisition.lvclass">)  [unwired: 7 in]
                n3530 = local read "Filter4"() -> (w7790:u8)
                n3531 = call-dynamic "Write Filter.vi"("error in (no error)"=w7787, "Filter"=w7790, "Channel in"=w7789) -> ("error out"=w7786:errorcluster, "Channel out"=w7788:refnum<class "Channel.lvclass">)  [unwired: 7 in]
                n3532 = call-dynamic "Read Interface.vi"("error in (no error)"=w7786, "Channel in"=w7788) -> ("error out"=w7799:errorcluster, "Interface.lvclass"=w7800:refnum<class "Interface.lvclass">, "Channel out"=w7812:refnum<class "Channel.lvclass">)  [unwired: 7 in]
                n3533 = call-dynamic "Write Suffix.vi"("error in (no error)"=w7799, "Suffix"=w7818, "Interface in"=w7800) -> ("error out"=w7817:errorcluster, "Interface out"=w7811:refnum<class "Interface.lvclass">)  [unwired: 7 in]
                n3534 = call-dynamic "Write ObsType.vi"("error in (no error)"=w7817, "ObsType"=w7803, "Interface in"=w7811) -> ("error out"=w7816:errorcluster, "Interface out"=w7810:refnum<class "Interface.lvclass">)  [unwired: 7 in]
                n3535 = call-dynamic "Write Object.vi"("error in (no error)"=w7816, "Object"=w7802, "Interface in"=w7810) -> ("error out"=w7815:errorcluster, "Interface out"=w7809:refnum<class "Interface.lvclass">)  [unwired: 7 in]
                n3536 = call-dynamic "Write Comments.vi"("error in (no error)"=w7815, "Comments"=w7804, "Interface in"=w7809) -> ("error out"=w7798:errorcluster, "Interface out"=w7797:refnum<class "Interface.lvclass">)  [unwired: 7 in]
                n3537 = call-dynamic "Write Observer.vi"("error in (no error)"=w7798, "Observer"=w7801, "Interface in"=w7797) -> ("error out"=w7796:errorcluster, "Interface out"=w7795:refnum<class "Interface.lvclass">)  [unwired: 7 in]
                n3538 = call-dynamic "Write Interface.vi"("error in (no error)"=w7796, "Interface.lvclass"=w7795, "Channel in"=w7812) -> ("error out"=w7792:errorcluster, "Channel out"=w7794:refnum<class "Channel.lvclass">)  [unwired: 7 in]
                n3539 = disable-structure shown="Enabled" {
                  disable-tunnel: w7794 -> [w7829 w7834]
                  disable-tunnel: [w7827 w7834] -> w7793
                  disable-tunnel: w7792 -> [w7826 w7833]
                  disable-tunnel: [w7825 w7833] -> w7791
                  frame Disabled {
                    n3540 = call-dynamic "Read State Machine.vi"("error in (no error)"=w7826, "Device in"=w7829) -> ("error out"=w7832:errorcluster, "State Machine.lvclass"=w7824:refnum<class "State Machine.lvclass">, "Device out"=w7828:refnum<class "Channel.lvclass">)  [unwired: 7 in]
                    n3541 = call "Next State.vi"("error in (no error)"=w7832, "New_State"=12, "State Machine in"=w7824) -> ("error out"=w7831:errorcluster, "State Machine out"=w7823:refnum<class "State Machine.lvclass">)  [unwired: 7 in]
                    n3542 = call-dynamic "Write State Machine.vi"("error in (no error)"=w7831, "State Machine.lvclass"=w7823, "Device in"=w7828) -> ("error out"=w7825:errorcluster, "Device out"=w7827:refnum<class "Channel.lvclass">)  [unwired: 7 in]
                  }
                  frame Enabled {
                  }
                }
                n3543 = call-dynamic "Write Channel.vi"("error in (no error)"=w7791, "Channel.lvclass"=w7793, "Acquisition in"=w7807) -> ("error out"=w7805:errorcluster, "Acquisition out"=w7806:refnum<class "Acquisition.lvclass">)  [unwired: 7 in]
                n3544 = call-dynamic "Write AcquisitionD.vi"("error in (no error)"=w7805, "Acquisition.lvclass"=w7806, "S4ACS_GUI in"=w7808) -> ("error out"=w7819:errorcluster, "S4ACS_GUI out"=w7820:refnum<class "S4GUI.lvclass">)  [unwired: 7 in]
              }
            }
          }
          frame Enabled {
          }
        }
      }
      event "Observer": Value Change {
        n3545 = event-data() -> ("NewVal"=w7867:string)  [unwired: 1 in, 5 out]
        n3546 = disable-structure shown="Disabled" {
          disable-tunnel: w7870 -> [w7885 w7886]
          disable-tunnel: w7867 -> [w7884 _]
          disable-tunnel: [w7883 w7886] -> w7869
          frame Disabled {
            n3547 = String Length(string=w7884) -> (length=w7882:i32)
            n3548 = Equal To 0?(x=w7882) -> (x = 0?=w7881:bool)
            n3549 = Select(t=u32 16777216, s=w7881, f=u32 16777225) -> (s? t:f=w7879:u32)
            n3550 = property on="Observer" class="Str"(error in=w7885, "Text.BGColor"=w7879) -> (error out=w7883:errorcluster)  [unwired: 1 in, 1 out]
          }
          frame Enabled {
            # "Não se usa mais o texto de fundo\ndo controle \"Observer\""
          }
        }
        n3551 = case shown="False" FALSE {
          tunnel: w7877 -> [w7895 w8133]
          tunnel: w7876 -> [w7894 _]
          tunnel: w7875 -> [w7893 _]
          tunnel: w7874 -> [w7892 _]
          tunnel: w7867 -> [w7891 _]
          tunnel: w7873 -> [w7890 _]
          tunnel: [w7889 w8133] -> w7872
          tunnel: [w7888 w8132] -> w7871
          tunnel: w7869 -> [w7887 w8132]
          frame False {
            n3552 = stacked-sequence {
              seq-local: [w7915 _ _ _] -> [_ w7985 _ _]
              seq-local: [w7914 _ _ _] -> [_ w7984 _ _]
              seq-local: [_ w7983 _ _] -> [_ _ w8044 _]
              seq-local: [_ w7982 _ _] -> [_ _ w8043 _]
              seq-local: [_ _ w8042 _] -> [_ _ _ w8103]
              seq-local: [_ _ w8041 _] -> [_ _ _ w8102]
              tunnel: w7887 -> [w7925 _ _ _]
              tunnel: w7895 -> [w7924 _ _ _]
              tunnel: [_ _ _ w8101] -> w7889
              tunnel: [_ _ _ w8100] -> w7888
              tunnel: w7893 -> [w7913 w7981 w8040 w8099]
              tunnel: w7892 -> [w7912 w7980 w8030 w8089]
              tunnel: w7890 -> [w7911 w7970 w8029 w8088]
              tunnel: w7894 -> [w7910 w7969 w8028 w8087]
              tunnel: w7891 -> [w7909 w7968 w8027 w8086]
              frame #0 {
                # "suffix"
                n3553 = call-dynamic "Read AcquisitionA.vi"("error in (no error)"=w7925, "S4ACS_GUI in"=w7924) -> ("error out"=w7923:errorcluster, "Acquisition.lvclass"=w7922:refnum<class "Acquisition.lvclass">, "S4ACS_GUI out"=w7919:refnum<class "S4GUI.lvclass">)  [unwired: 7 in]
                n3554 = call-dynamic "Read Channel.vi"("error in (no error)"=w7923, "Acquisition in"=w7922) -> ("error out"=w7897:errorcluster, "Channel.lvclass"=w7900:refnum<class "Channel.lvclass">, "Acquisition out"=w7918:refnum<class "Acquisition.lvclass">)  [unwired: 7 in]
                n3555 = local read "Filter1"() -> (w7898:u8)
                n3556 = call-dynamic "Write Filter.vi"("error in (no error)"=w7897, "Filter"=w7898, "Channel in"=w7900) -> ("error out"=w7896:errorcluster, "Channel out"=w7899:refnum<class "Channel.lvclass">)  [unwired: 7 in]
                n3557 = call-dynamic "Read Interface.vi"("error in (no error)"=w7896, "Channel in"=w7899) -> ("error out"=w7907:errorcluster, "Interface.lvclass"=w7908:refnum<class "Interface.lvclass">, "Channel out"=w7921:refnum<class "Channel.lvclass">)  [unwired: 7 in]
                n3558 = call-dynamic "Write Suffix.vi"("error in (no error)"=w7907, "Suffix"=w7913, "Interface in"=w7908) -> ("error out"=w7926:errorcluster, "Interface out"=w7920:refnum<class "Interface.lvclass">)  [unwired: 7 in]
                n3559 = disable-structure shown="Enabled" {
                  disable-tunnel: w7926 -> [w7940 w7941]
                  disable-tunnel: w7920 -> [w7937 w7942]
                  disable-tunnel: w7912 -> [w7934 _]
                  disable-tunnel: w7911 -> [w7933 _]
                  disable-tunnel: w7910 -> [w7932 _]
                  disable-tunnel: w7909 -> [w7931 _]
                  disable-tunnel: [w7928 w7942] -> w7906
                  disable-tunnel: [w7927 w7941] -> w7905
                  frame Disabled {
                    # "observer"
                    # "comment"
                    # "object"
                    # "obsType"
                    n3560 = call-dynamic "Write ObsType.vi"("error in (no error)"=w7940, "ObsType"=w7933, "Interface in"=w7937) -> ("error out"=w7939:errorcluster, "Interface out"=w7936:refnum<class "Interface.lvclass">)  [unwired: 7 in]
                    n3561 = call-dynamic "Write Object.vi"("error in (no error)"=w7939, "Object"=w7932, "Interface in"=w7936) -> ("error out"=w7938:errorcluster, "Interface out"=w7935:refnum<class "Interface.lvclass">)  [unwired: 7 in]
                    n3562 = call-dynamic "Write Comments.vi"("error in (no error)"=w7938, "Comments"=w7934, "Interface in"=w7935) -> ("error out"=w7930:errorcluster, "Interface out"=w7929:refnum<class "Interface.lvclass">)  [unwired: 7 in]
                    n3563 = call-dynamic "Write Observer.vi"("error in (no error)"=w7930, "Observer"=w7931, "Interface in"=w7929) -> ("error out"=w7927:errorcluster, "Interface out"=w7928:refnum<class "Interface.lvclass">)  [unwired: 7 in]
                  }
                  frame Enabled {
                  }
                }
